vi "AM-sinal-modulation.vi"() -> ()   [LabVIEW 2013]
panel:
  out "CP":dbl caption="Constante de proporcionalidade(K)"
  in  "m":dbl(slide)=0.001 caption="Índice de modulação (m)" min=0.0 max=1.0 step=0.01 scale=0.0..1.0
  in  "N":dbl=1.0 caption="Numero de ciclos" format="%#_13g"
  out "mod":cluster{i32[], dbl[]}(graph) caption="Modulação"
  out "Portadora":cluster{i32[], dbl[]}(graph)
  out "Informação":cluster{i32[], dbl[]}(graph)
  in  "Nc":dbl caption="Precisao temporal"
  in  "fm":dbl caption="Frequencia do sinal modulador"
  in  "fp":dbl caption="Frequencia da portadora"
  in  "E0":dbl caption="Amplitude da portadora"
  in  "Em":dbl caption="Amplitude do sinal modulador"
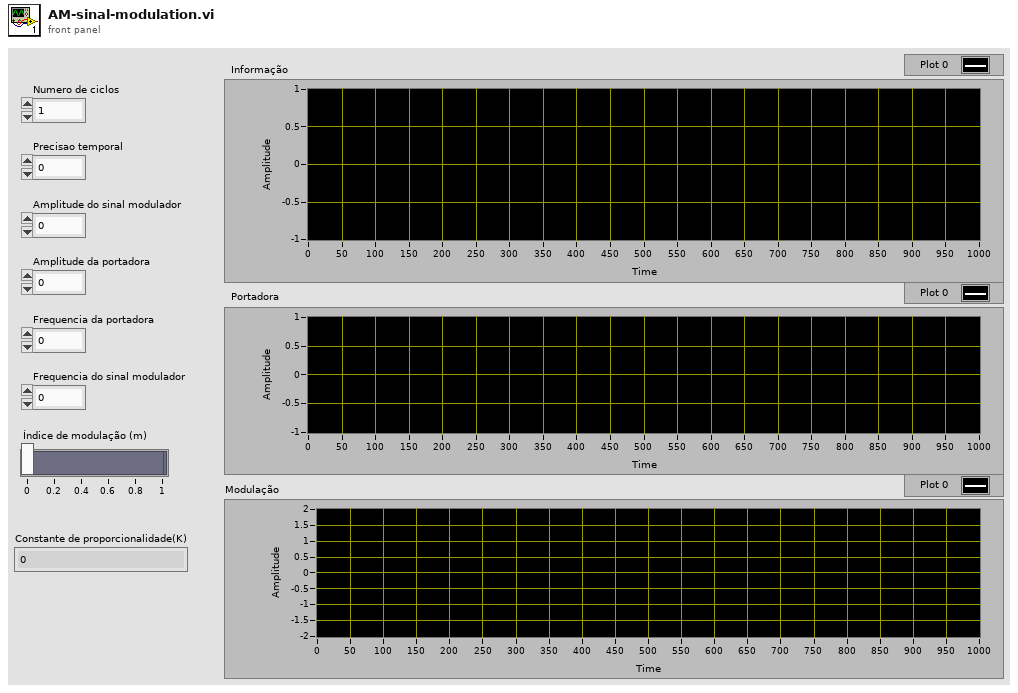
[diagram p1: front panel]
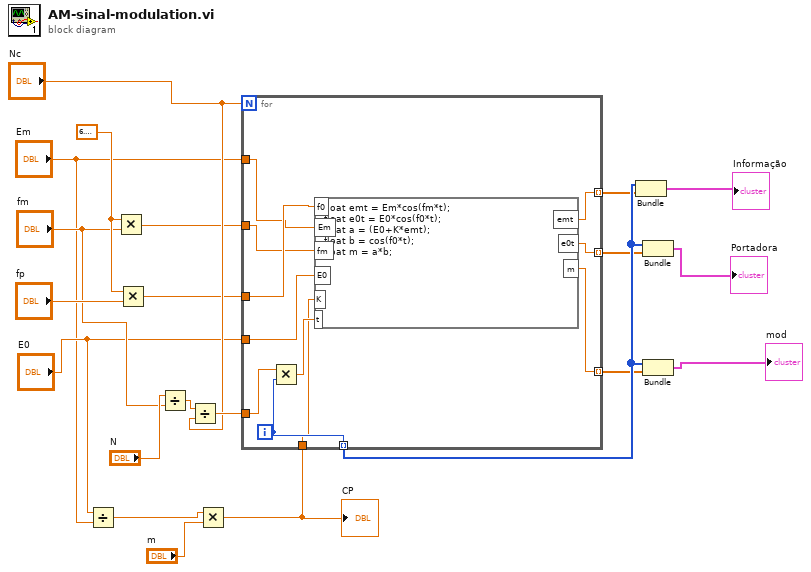
[diagram p0: block diagram]
diagram:
  w21 = 6.283185307179586
  n1 = Divide(x="E0", y="Em") -> (x/y=w2:dbl)
  n2 = Multiply(x=w21, y="fm") -> (x*y=w14:dbl)
  n3 = Multiply(x=w21, y="fp") -> (x*y=w15:dbl)
  n4 = Divide(x="N", y="fm") -> (x/y=w18:dbl)
  n5 = Divide(x=w18, y="Nc") -> (x/y=w17:dbl)
  n6 = Multiply(x=w2, y="m") -> (x*y=w1:dbl)
  "CP" <- w1
  n7 = for {
    N: "Nc" -> [_]
    tunnel: "Em" -> [w25]
    tunnel: "E0" -> [w26]
    tunnel: w14 -> [w27]
    tunnel: w15 -> [w28]
    tunnel: [w31] -> w12 mode=indexing
    tunnel: w17 -> [w32]
    tunnel: w1 -> [w29]
    tunnel: [w24] -> w11 mode=indexing
    tunnel: [w23] -> w10 mode=indexing
    tunnel: [w22] -> w9 mode=indexing
    i -> [w31]
    n8 = Multiply(x=w32, y=w31) -> (x*y=w30:dbl)
    n9 = formula code="float emt = Em*cos(fm*t);\nfloat e0t = E0*cos(f0*t);\nfloat a = (E0+K*emt);\nfloat b = cos(f0*t);\nfloat m = a*b;"("fm"=w27, "f0"=w28, "Em"=w25, "E0"=w26, "t"=w30, "K"=w29) -> ("emt"=w24:dbl, "e0t"=w23:dbl, "m"=w22:dbl)
  }
  n10 = Bundle(w12, w11) -> (→"Informação":cluster{i32[], dbl[]})  [unwired: 1 in]
  n11 = Bundle(w12, w10) -> (→"Portadora":cluster{i32[], dbl[]})  [unwired: 1 in]
  n12 = Bundle(w12, w9) -> (→"mod":cluster{i32[], dbl[]})  [unwired: 1 in]
